vi "CreatFromSerialNum.vi"(8 "error in (no error)":errorcluster, 11 "APD Serial #":string) -> (0 "error out":errorcluster, 3 "APDClass out":refnum<class "APDClass.lvclass">)   [LabVIEW 2020, in "APDClass.lvclass"]
uses:
  APDClass.lvclass
  iRFData.ctl
  GainData.ctl
panel:
  out "GainRawTempError":errorcluster
  out "GainData":T1
  out "Mesurment date":string
  out "iRF Data":T2
  out "Waveform Graph":dbl[][](graph)
  out "Gain Curve":cluster{dbl[], dbl[]}(graph)
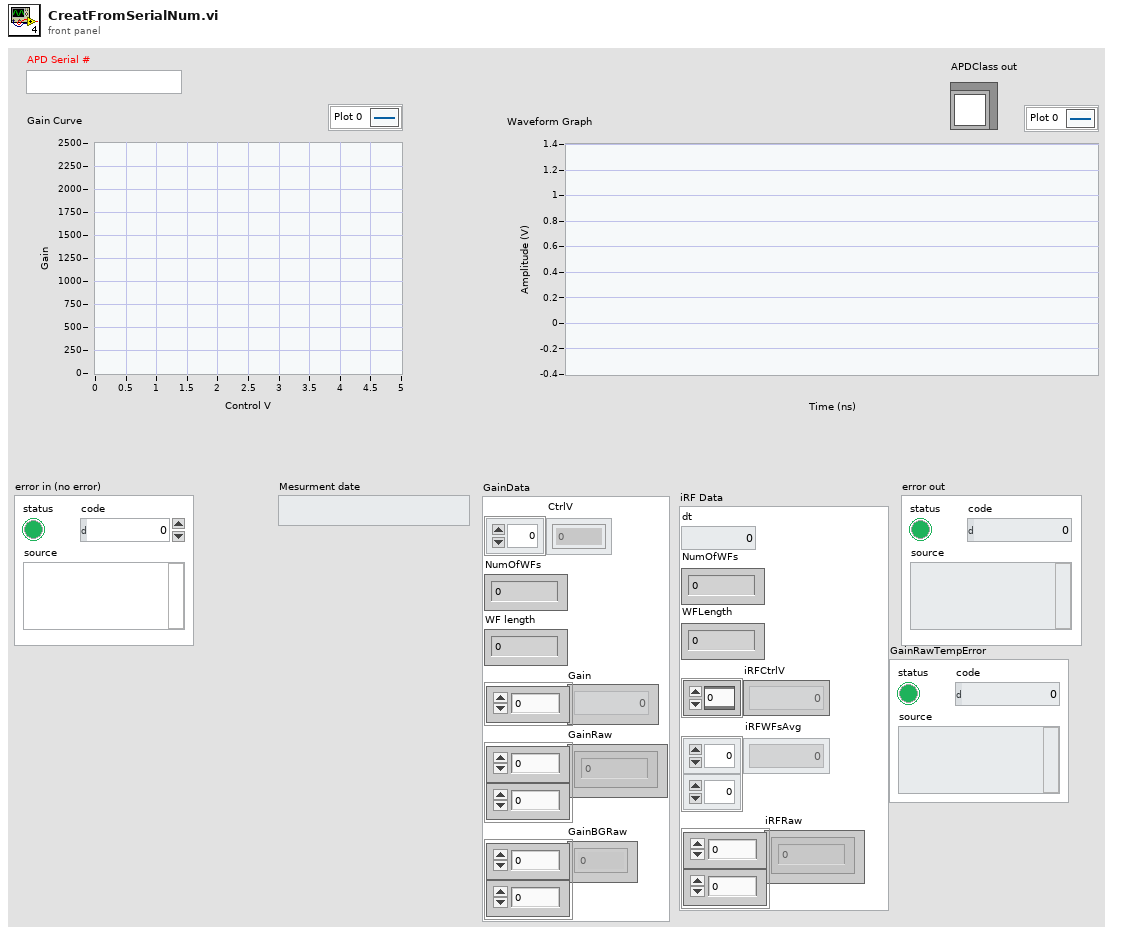
[diagram p1: front panel]
types:
  T1 = typedef "GainData.ctl" = cluster{"CtrlV":dbl[], "NumOfWFs":i32, "WF length":i32, "Gain":dbl[], "GainRaw":dbl[][], "GainBGRaw":dbl[][]}
  T2 = typedef "iRFData.ctl" = cluster{"dt":dbl, "NumOfWFs":i32, "WFLength":i32, "iRFCtrlV":dbl[], "iRFWFsAvg":dbl[][], "iRFRaw":dbl[][]}
  T3 = enum16{"open", "open or create", "create or replace", "create", "open (read-only)"}
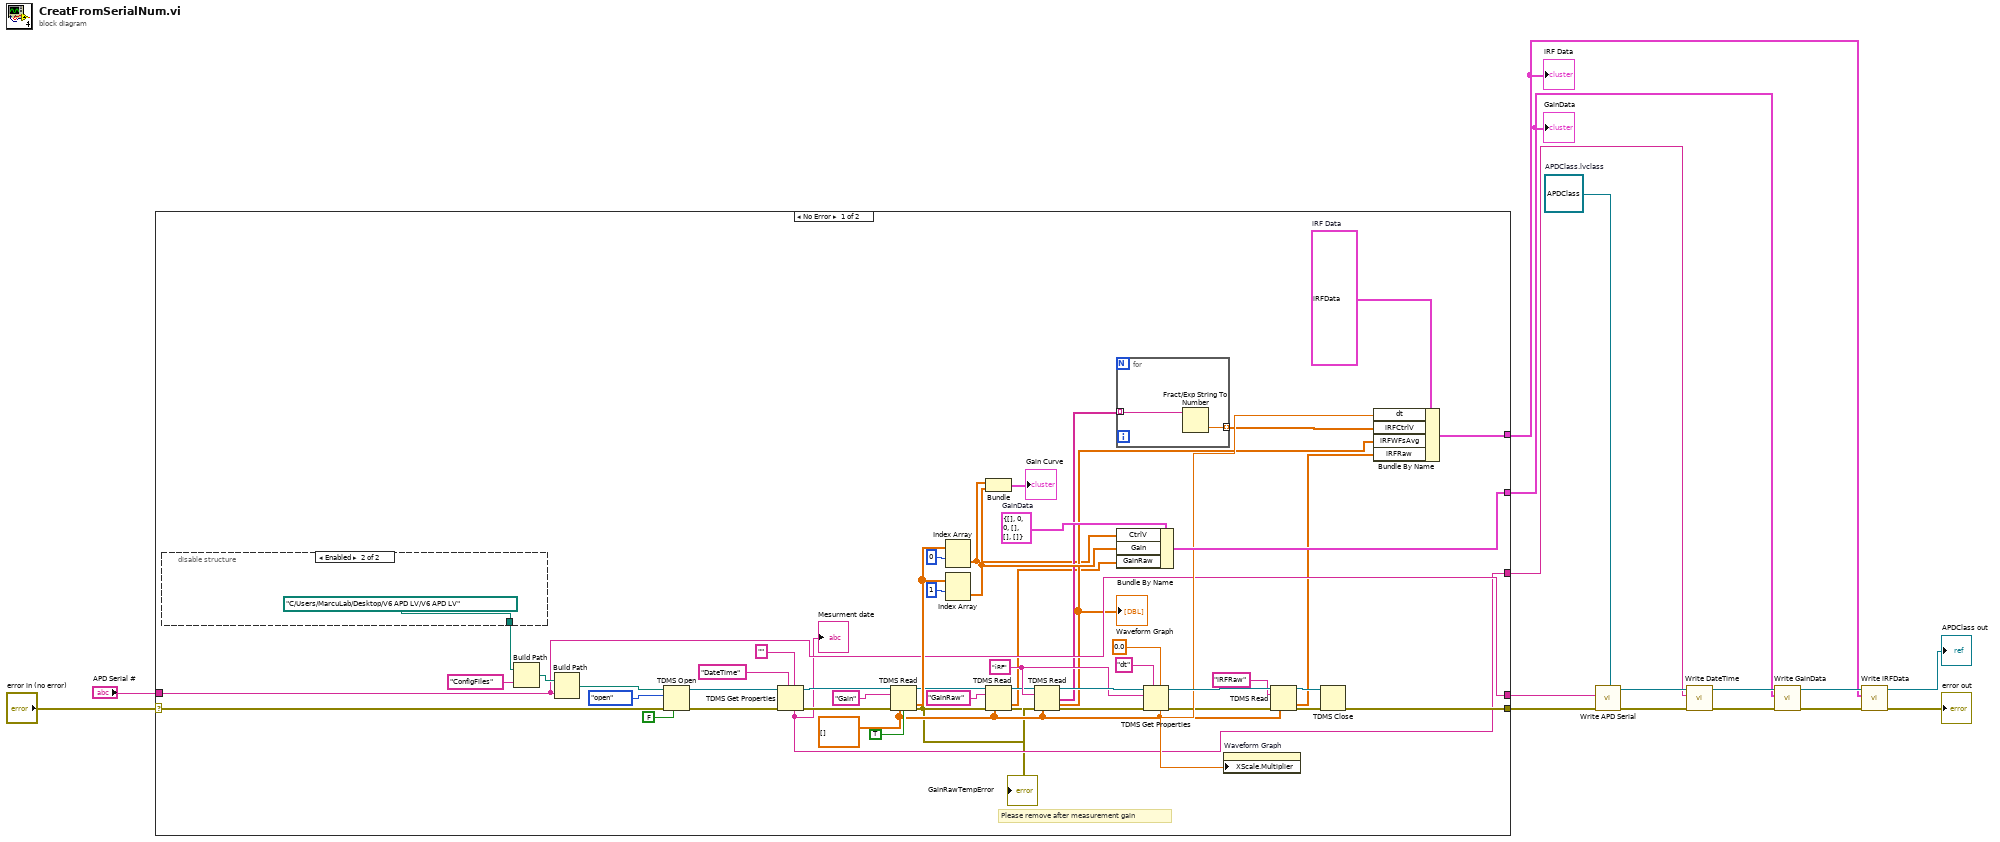
[diagram p0: block diagram]
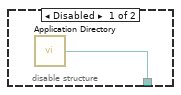
[diagram p2: hidden frame]
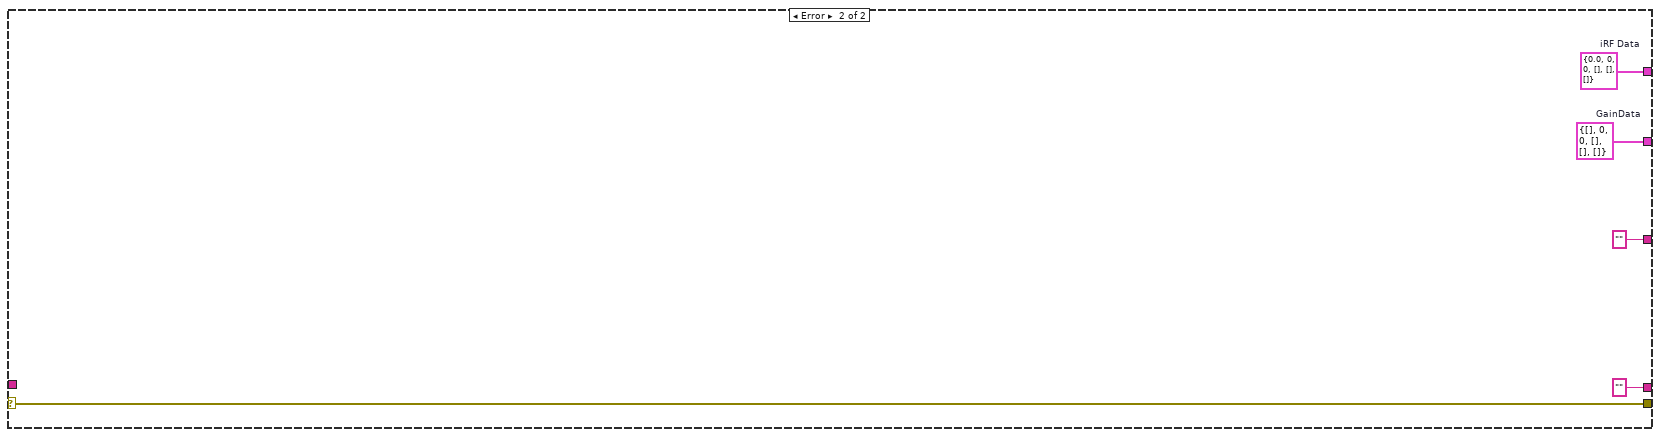
[diagram p3: hidden frame]
diagram:
  w14 = refnum<class "APDClass.lvclass"> refnum  # APDClass.lvclass
  n1 = case shown="No Error" "error in (no error)" {
    selector: "error in (no error)" -> [w45 w75]
    tunnel: [w44 w75] -> w12
    tunnel: "APD Serial #" -> [w40 _]
    tunnel: [w43 w74] -> w10
    tunnel: [w42 w71] -> w1
    tunnel: [w40 "" ("APD Serial #")] -> w13
    tunnel: [w33 ""] -> w2
    frame No Error {
      w32 = T1 {"CtrlV"=[], "NumOfWFs"=0, "WF length"=0, "Gain"=[], "GainRaw"=[], "GainBGRaw"=[]}  # GainData
      w50 = T2 {"dt"=0.0, "NumOfWFs"=0, "WFLength"=0, "iRFCtrlV"=[0.0, 0.1, 0.2, 0.30000000000000004, 0.4, 0.5, 0.6000000000000001, 0.7000000000000001, 0.8, 0.9, 1.0, 1.1, 1.2000000000000002, 1.3, 1.4000000000000001, 1.5, 1.6, 1.7000000000000002, 1.8, 1.9000000000000001, 2.0, 2.1, 2.2, 2.3000000000000003, 2.4000000000000004, 2.5, 2.6, 2.7, 2.8000000000000003, 2.9000000000000004, 3.0, 3.1, 3.2, 3.3000000000000003, 3.4000000000000004, 3.5, 3.6, 3.7, 3.8000000000000003, 3.9000000000000004, 4.0, 4.1000000000000005, 4.2, 4.3, 4.4, 4.5, 4.6000000000000005], "iRFWFsAvg"=array47x600[28200 elements], "iRFRaw"=[]}  # iRF Data
      w48 = "iRF" ("group name in (Untitled)")
      w20 = dbl[][] []
      # "Please remove after measurement gain"
      n2 = disable-structure shown="Enabled" {
        disable-tunnel: [w67 path "C:/Users/MarcuLab/Desktop/V6 APD LV/V6 APD LV" ("Application Directory")] -> w66
        frame Disabled {
          n3 = call <vilib>:"Application Directory.vi"() -> ("Application Directory"=w67:path)
        }
        frame Enabled {
        }
      }
      n4 = Build Path(base path=w66, name or relative path="ConfigFiles") -> (appended path=w64:path)
      n5 = Build Path(base path=w64, name or relative path=w40) -> (appended path=w63:path)
      n6 = TDMS Open(6:FALSE ("disable buffering? (T)"), 8:w45, 10:T3."open" ("operation (0:open)"), 11:w63) -> (0:w38:errorcluster, 3:w39:refnum<k34>)  [unwired: 3 in]
      n7 = TDMS Get Properties(5:"", 7:"DateTime" ("property name"), 8:w38, 11:w39) -> (0:w34:errorcluster, 3:w35:refnum<k34>, 4:w33:string)  [unwired: 2 in, 3 out]
      "Mesurment date" <- w33
      n8 = TDMS Read(0:w35, 5:"Gain" ("group name in"), 11:w34, 12:w20, 13:TRUE ("return channels in file order? (F)")) -> (4:w54:refnum<k34>, 10:w57:dbl[][], 15:w18:errorcluster)  [unwired: 3 in, 3 out]
      n9 = Index Array(array=w57, index (row)=0) -> (element=w28:dbl[])  [unwired: 1 in]
      n10 = Index Array(array=w57, index (row)=1) -> (element=w51:dbl[])  [unwired: 1 in]
      n11 = Bundle(w28, w51) -> (→"Gain Curve":cluster{dbl[], dbl[]})  [unwired: 1 in]
      n12 = TDMS Read(0:w54, 5:"GainRaw" ("group name in (Untitled)"), 11:w18, 12:w20) -> (4:w27:refnum<k34>, 10:w25:dbl[][], 15:→"GainRawTempError":errorcluster)  [unwired: 4 in, 3 out]
      n13 = TDMS Read(0:w27, 5:w48, 11:w18, 12:w20) -> (4:w53:refnum<k34>, 8:w31:string[], 10:w30:dbl[][], 15:w52:errorcluster)  [unwired: 4 in, 2 out]
      "Waveform Graph" <- w30
      n14 = for {
        tunnel: w31 -> [w70] mode=indexing
        tunnel: [w69] -> w29 mode=indexing
        n15 = Fract/Exp String To Number(string=w70) -> (number=w69:dbl)  [unwired: 3 in, 1 out]
      }
      n16 = Bundle By Name(cluster=w32, "CtrlV"=w28, "Gain"=w51, "GainRaw"=w25) -> (w42:T1)
      n17 = TDMS Get Properties(5:0.0, 7:"dt", 8:w52, 10:w48, 11:w53) -> (0:w23:errorcluster, 3:w49:refnum<k34>, 4:w41:dbl)  [unwired: 1 in, 3 out]
      n18 = property on="Waveform Graph" class="WFGraph (strict)"("XScale.Multiplier"=w41) -> ()  [unwired: 2 in, 2 out]
      n19 = TDMS Read(0:w49, 5:"iRFRaw" ("group name"), 11:w23, 12:w20) -> (4:w24:refnum<k34>, 10:w19:dbl[][], 15:w22:errorcluster)  [unwired: 4 in, 3 out]
      n20 = TDMS Close(8:w22, 11:w24) -> (0:w44:errorcluster)  [unwired: 1 out]
      n21 = Bundle By Name(cluster=w50, "dt"=w41, "iRFCtrlV"=w29, "iRFWFsAvg"=w30, "iRFRaw"=w19) -> (w43:T2)
    }
    frame Error {
      w71 = T1 {"CtrlV"=[], "NumOfWFs"=0, "WF length"=0, "Gain"=[], "GainRaw"=[], "GainBGRaw"=[]}  # GainData
      w74 = T2 {"dt"=0.0, "NumOfWFs"=0, "WFLength"=0, "iRFCtrlV"=[], "iRFWFsAvg"=[], "iRFRaw"=[]}  # iRF Data
    }
  }
  "iRF Data" <- w10
  "GainData" <- w1
  n22 = call-dynamic "Write APD Serial.vi"("error in (no error)"=w12, "APD Serial #"=w13, "APDClass in"=w14) -> ("error out"=w5:errorcluster, "APDClass out"=w6:refnum<class "APDClass.lvclass">)  [unwired: 7 in]
  n23 = call-dynamic "Write DateTime.vi"("error in (no error)"=w5, "DateTime"=w2, "APDClass in"=w6) -> ("error out"=w3:errorcluster, "APDClass out"=w4:refnum<class "APDClass.lvclass">)  [unwired: 7 in]
  n24 = call-dynamic "Write GainData.vi"("error in (no error)"=w3, "GainData"=w1, "APDClass in"=w4) -> ("error out"=w9:errorcluster, "APDClass out"=w11:refnum<class "APDClass.lvclass">)  [unwired: 7 in]
  n25 = call-dynamic "Write iRFData.vi"("error in (no error)"=w9, "iRFData"=w10, "APDClass in"=w11) -> ("error out"=→"error out":errorcluster, "APDClass out"=→"APDClass out":refnum<class "APDClass.lvclass">)  [unwired: 7 in]
